vi "QuadRotor_Monitoring_LV1.vi"() -> ()   [LabVIEW 2015]
uses:
  <vilib>/Instr/_visa.llb/VISA Set IO Buffer Mask.ctl
  <vilib>/Instr/_visa.llb/VISA Configure Serial Port (Instr).vi
panel:
  in  "Lontitude_W3":i32=1005738310
  in  "Latitude_W3":i32=139458720
  in  "Lontitude_W2":i32=1005738310
  in  "Latitude_W2":i32=139458720
  in  "Lontitude_W1":i32=1005738310
  in  "Latitude_W1":i32=139458720
  in  "Lon_home":i32=1005748870
  in  "Lat_home":i32=139456050
  out "(GPS_numSat)":u16
  out "return count 2":u32
  out "Roob":i32
  out "Altitude_(Auto)":ext format="%#_3g"
  in  "Set_Altitude_(Auto)":dbl=2.5
  out "string":string
  out "Mode":ext format="%.2f"
  out "Altitude":dbl(slide) scale=0.0..20.0
  out "Altitude":ext format="%.2f"
  out "Yaw":dbl(knob) scale=-180.0..180.0
  out "Pitch":dbl(knob) scale=-90.0..90.0
  out "Roll":dbl(knob) scale=-90.0..90.0
  in  "Write to Quad":bool
  out "Header_58":u8
  out "GPS_Longtitude":ext format="%#.7f"
  out "Pitch":ext format="%.2f"
  out "Yaw":ext format="%.2f"
  out "GPS_Latitude":ext format="%#.7f"
  out "Roll":ext format="%.2f"
  out "return count":u32
  in  "stop":bool
  in  "VISA Serial Data":refnum<visa-resource-name>
  # "Quad Rotor Monitoring and Control with GPS Waypoint"
  # "Data Write to Autonomous Quad Rotor (LAT 9 Point), (LON 10 Point) with Google Map tracking Navigator"
  # "Ex  13.8591411 = 138591411 , 100.5231704 = 1005231704 Using in integer  I32"
  # "9 Point"
  # "10 Point"
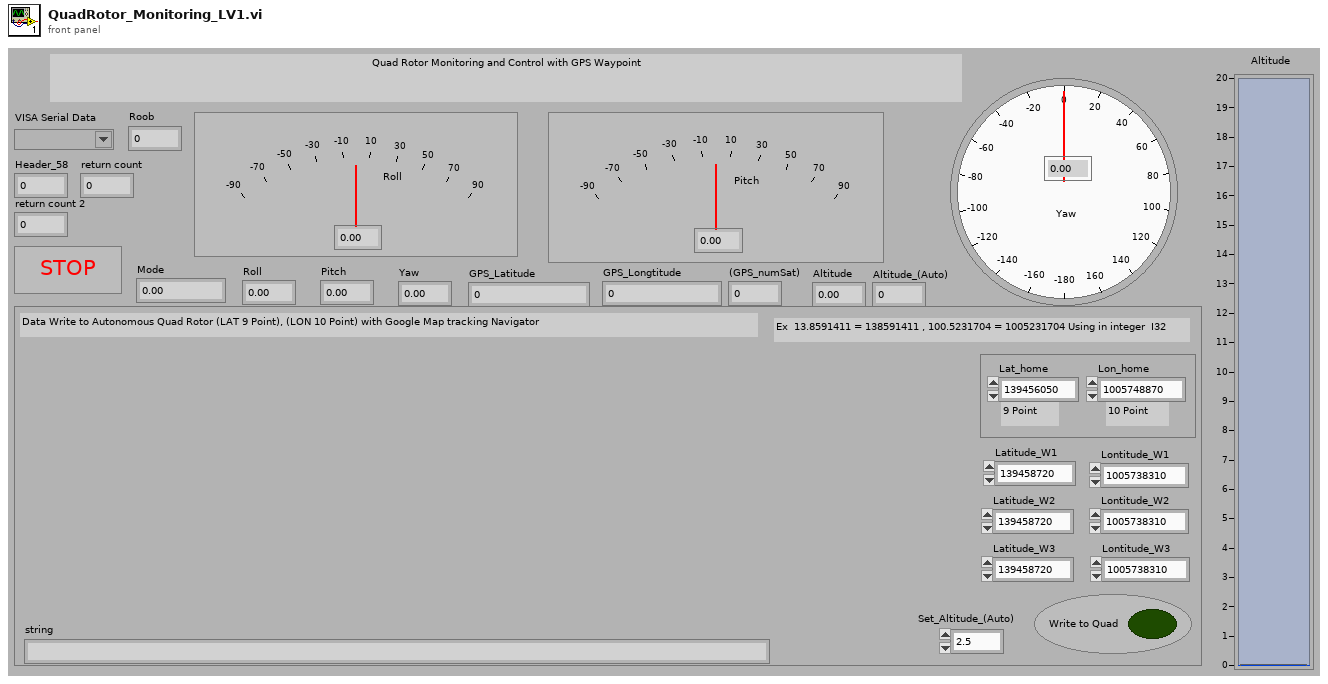
[diagram p1: front panel]
types:
  T1 = typedef "VISA Set IO Buffer Mask.ctl" = u16
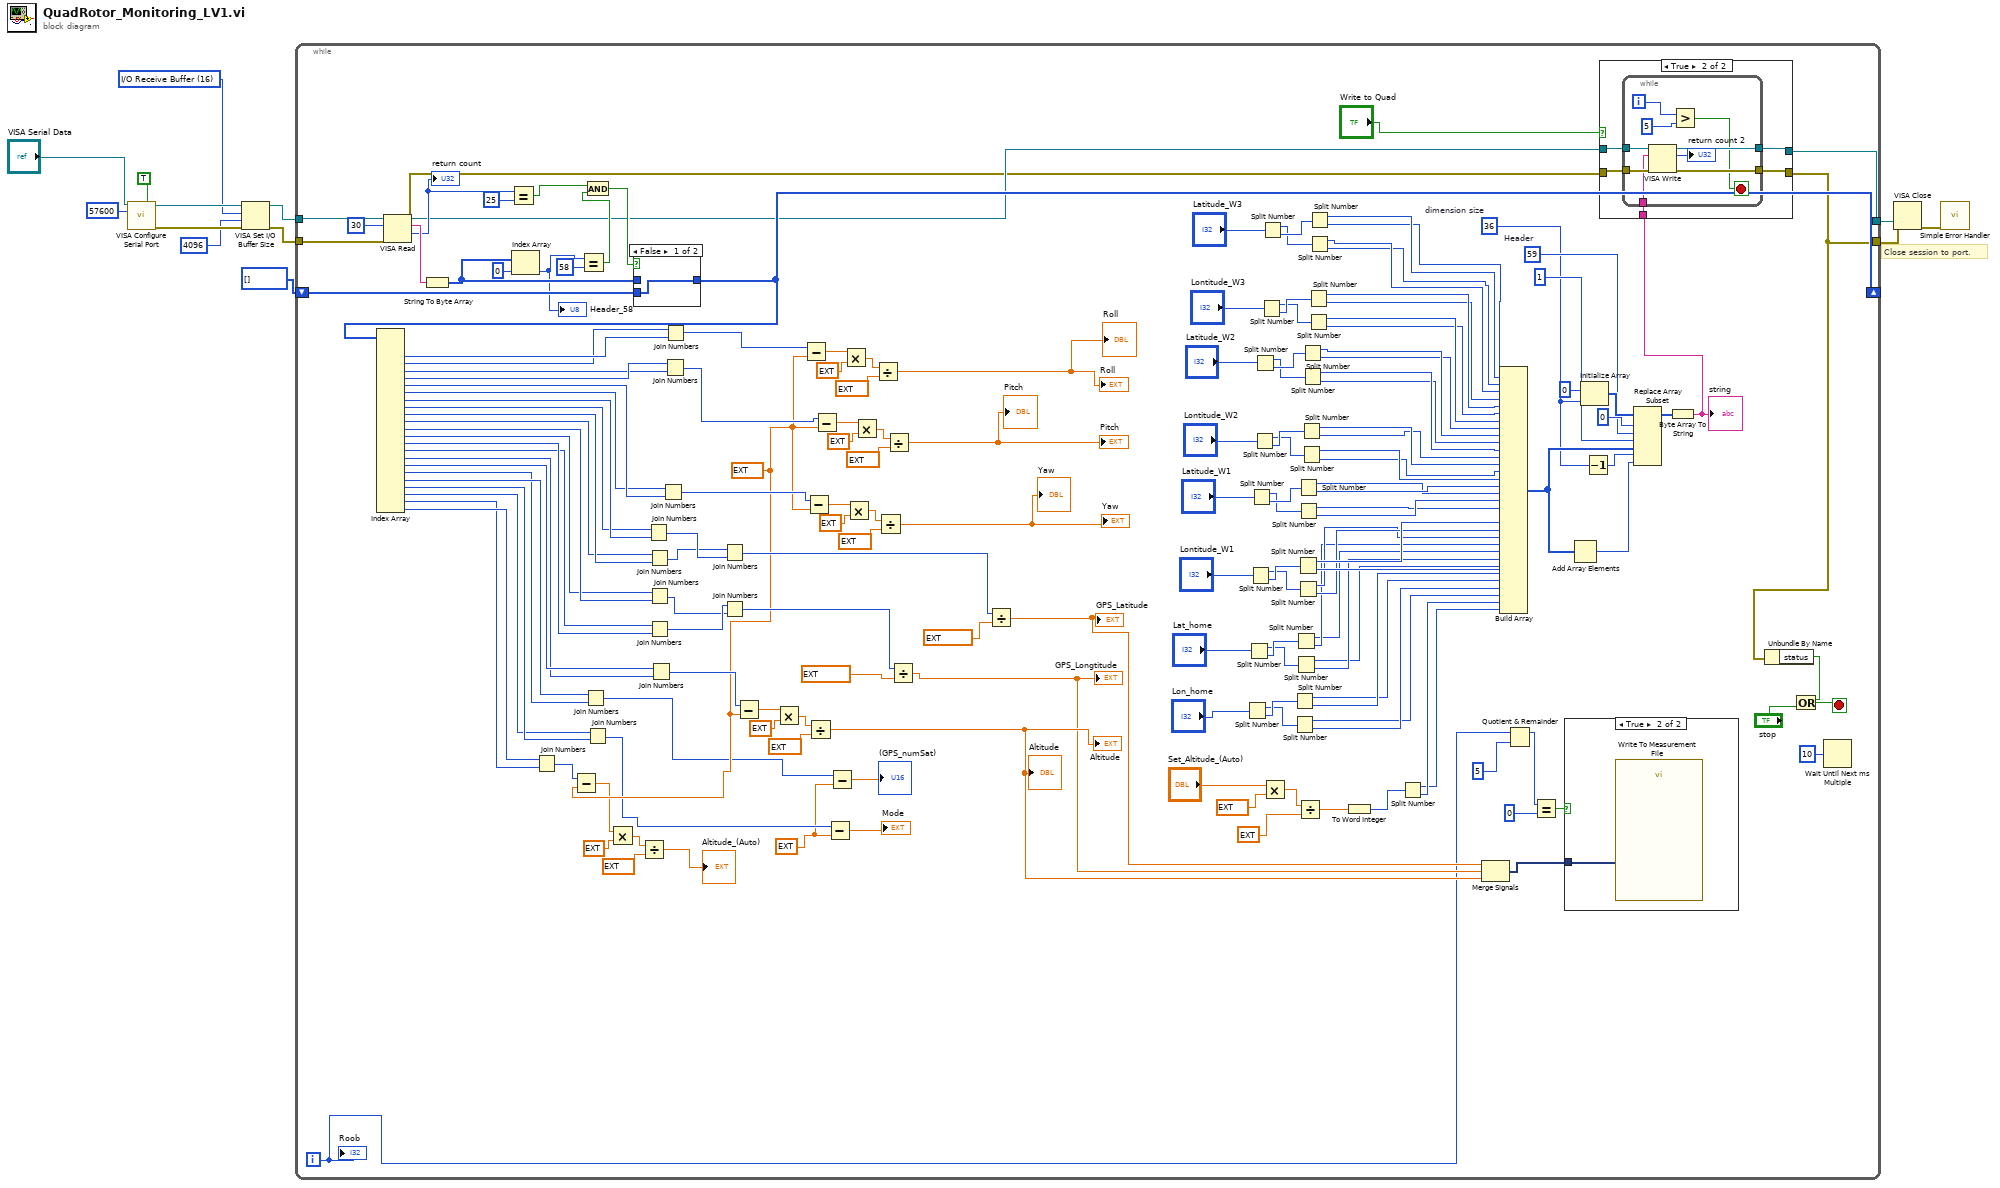
[diagram p0: block diagram]
diagram:
  w10 = T1 16 items=["I/O Receive Buffer"=16, "I/O Transmit Buffer"=32, "I/O Receive and Transmit Buffer"=48] ("Mask")
  # "Close session to port."
  n1 = call-poly "VISA Configure Serial Port"("VISA resource name"="VISA Serial Data", "Enable Termination\nChar (T)"=TRUE ("Enable Termination\nChar (T)"), "baud rate (9600)"=u32 57600) -> ("VISA resource name out"=w12:refnum<visa-resource-name>, "error out"=w11:errorcluster)  [unwired: 7 in, 4 out]
  n2 = VISA Set I/O Buffer Size(VISA resource name=w12, mask (16)=w10, size (4096)=u32 4096, error in (no error)=w11) -> (VISA resource name out=w8:refnum<visa-resource-name>, error out=w6:errorcluster)
  n3 = while {
    tunnel: [w142] -> w7
    tunnel: w8 -> [w183]
    tunnel: [w141] -> w5
    tunnel: w6 -> [w182]
    shift-right: [w152] -> _
    shift-left: u8[] [] ("unsigned byte array") -> [w153]
    i -> [w45]
    stop <- w186 stop-if-true
    w60 = 36  # dimension size
    w109 = u8 59  # Header
    w52 = ext 255.0 ("y")
    w70 = ext 32767.0 ("y")
    n4 = VISA Read(VISA resource name=w183, byte count=u32 30, error in (no error)=w182) -> (VISA resource name out=w144:refnum<visa-resource-name>, read buffer=w156:string, return count=w149:u32, error out=w143:errorcluster)
    "return count" <- w149
    n5 = String To Byte Array(string=w156) -> (unsigned byte array=w154:u8[])
    n6 = Equal?(x=w149, y=u32 25) -> (x = y?=w147:bool)
    n7 = Index Array(array=w154, index=0) -> (element=w146:u8)
    "Header_58" <- w146
    n8 = Equal?(x=w146, y=u8 58) -> (x = y?=w151:bool)
    n9 = And(x=w147, y=w151) -> (x .and. y?=w150:bool)
    n10 = case shown="False" w150 {
      tunnel: w154 -> [_ w205]
      tunnel: [w204 w205] -> w152
      tunnel: w153 -> [w204 _]
      frame False {
      }
      frame True {
      }
    }
    n11 = Index Array(array=w152) -> (element #2=w176:u8, element #3=w175:u8, element #4=w173:u8, element #5=w174:u8, element #6=w180:u8, element #7=w179:u8, element #8=w178:u8, element #9=w177:u8, element #10=w137:u8, element #11=w136:u8, element #12=w133:u8, element #13=w132:u8, element #14=w131:u8, element #15=w130:u8, element #16=w120:u8, element #17=w126:u8, element #18=w118:u8, element #19=w119:u8, element #20=w117:u8, element #21=w116:u8, element #22=w72:u8, element #23=w73:u8)  [unwired: 23 in, 1 out]
    n12 = Join Numbers(hi=w73, lo=w72) -> ((hi.lo)=w71:u16)
    n13 = Subtract(x=w71, y=w70) -> (x-y=w66:ext)
    n14 = Join Numbers(hi=w119, lo=w118) -> ((hi.lo)=w51:u16)
    n15 = Join Numbers(hi=w116, lo=w117) -> ((hi.lo)=w55:u16)
    n16 = Multiply(x=w66, y=ext 100.0) -> (x*y=w68:ext)
    n17 = Divide(x=w68, y=ext 32767.0) -> (x/y=→"Altitude_(Auto)":ext)
    n18 = Join Numbers(hi=w177, lo=w178) -> ((hi.lo)=w135:u16)
    n19 = Join Numbers(hi=w136, lo=w137) -> ((hi.lo)=w134:u16)
    n20 = Join Numbers(hi=w132, lo=w133) -> ((hi.lo)=w114:u16)
    n21 = Join Numbers(hi=w130, lo=w131) -> ((hi.lo)=w115:u16)
    n22 = Join Numbers(hi=w126, lo=w120) -> ((hi.lo)=w121:u16)
    n23 = Join Numbers(hi=w179, lo=w180) -> ((hi.lo)=w162:u16)
    n24 = Join Numbers(hi=w174, lo=w173) -> ((hi.lo)=w157:u16)
    n25 = Join Numbers(hi=w175, lo=w176) -> ((hi.lo)=w171:u16)
    n26 = Join Numbers(hi=w134, lo=w135) -> ((hi.lo)=w139:u32)
    n27 = Join Numbers(hi=w115, lo=w114) -> ((hi.lo)=w129:u32)
    n28 = Subtract(x=w121, y=w70) -> (x-y=w125:ext)
    n29 = Multiply(x=w125, y=ext 100.0) -> (x*y=w123:ext)
    n30 = Subtract(x=w171, y=w70) -> (x-y=w170:ext)
    n31 = Subtract(x=w162, y=w70) -> (x-y=w166:ext)
    n32 = Divide(x=w123, y=ext 32767.0) -> (x/y=w50:ext)
    "Altitude" <- w50
    "Altitude" <- w50
    n33 = Subtract(x=w157, y=w70) -> (x-y=w161:ext)
    n34 = Subtract(x=w55, y=w52) -> (x-y=→"Mode":ext)
    n35 = Subtract(x=w51, y=w52) -> (x-y=→"(GPS_numSat)":ext)
    n36 = Multiply(x=w170, y=ext 180.0) -> (x*y=w168:ext)
    n37 = Multiply(x=w166, y=ext 180.0) -> (x*y=w164:ext)
    n38 = Multiply(x=w161, y=ext 180.0) -> (x*y=w159:ext)
    n39 = Divide(x=w168, y=ext 32767.0) -> (x/y=→"Roll" →"Roll":ext)
    n40 = Divide(x=w164, y=ext 32767.0) -> (x/y=→"Yaw" →"Yaw":ext)
    n41 = Divide(x=w159, y=ext 32767.0) -> (x/y=→"Pitch" →"Pitch":ext)
    n42 = Divide(x=w129, y=ext 10000000.0) -> (x/y=w49:ext)
    "GPS_Longtitude" <- w49
    n43 = Divide(x=w139, y=ext 10000000.0) -> (x/y=w48:ext)
    "GPS_Latitude" <- w48
    n44 = Split Number(x="Lon_home") -> (hi(x)=w102:u16, lo(x)=w103:u16)
    n45 = Split Number(x="Lat_home") -> (hi(x)=w104:u16, lo(x)=w105:u16)
    n46 = Split Number(x="Lontitude_W1") -> (hi(x)=w106:u16, lo(x)=w107:u16)
    n47 = Split Number(x="Latitude_W1") -> (hi(x)=w84:u16, lo(x)=w85:u16)
    n48 = Split Number(x="Lontitude_W2") -> (hi(x)=w40:u16, lo(x)=w41:u16)
    n49 = Split Number(x="Latitude_W2") -> (hi(x)=w38:u16, lo(x)=w39:u16)
    n50 = Split Number(x="Lontitude_W3") -> (hi(x)=w34:u16, lo(x)=w35:u16)
    n51 = Split Number(x="Latitude_W3") -> (hi(x)=w32:u16, lo(x)=w33:u16)
    n52 = Multiply(x="Set_Altitude_(Auto)", y=ext 32767.0) -> (x*y=w76:ext)
    n53 = Split Number(x=w103) -> (hi(x)=w88:u8, lo(x)=w89:u8)
    n54 = Split Number(x=w102) -> (hi(x)=w86:u8, lo(x)=w87:u8)
    n55 = Split Number(x=w105) -> (hi(x)=w92:u8, lo(x)=w93:u8)
    n56 = Split Number(x=w104) -> (hi(x)=w90:u8, lo(x)=w91:u8)
    n57 = Split Number(x=w107) -> (hi(x)=w96:u8, lo(x)=w97:u8)
    n58 = Split Number(x=w106) -> (hi(x)=w94:u8, lo(x)=w95:u8)
    n59 = Split Number(x=w85) -> (hi(x)=w100:u8, lo(x)=w101:u8)
    n60 = Split Number(x=w84) -> (hi(x)=w98:u8, lo(x)=w99:u8)
    n61 = Divide(x=w76, y=ext 100.0) -> (x/y=w74:ext)
    n62 = Split Number(x=w41) -> (hi(x)=w27:u8, lo(x)=w26:u8)
    n63 = Split Number(x=w40) -> (hi(x)=w29:u8, lo(x)=w28:u8)
    n64 = Split Number(x=w39) -> (hi(x)=w23:u8, lo(x)=w22:u8)
    n65 = Split Number(x=w38) -> (hi(x)=w25:u8, lo(x)=w24:u8)
    n66 = Split Number(x=w35) -> (hi(x)=w19:u8, lo(x)=w18:u8)
    n67 = Split Number(x=w34) -> (hi(x)=w21:u8, lo(x)=w20:u8)
    n68 = Split Number(x=w33) -> (hi(x)=w15:u8, lo(x)=w14:u8)
    n69 = Split Number(x=w32) -> (hi(x)=w17:u8, lo(x)=w16:u8)
    n70 = To Word Integer(number=w74) -> (16bit integer=w77:i16)
    n71 = Split Number(x=w77) -> (hi(x)=w78:u8, lo(x)=w79:u8)
    n72 = Merge Signals(w48, w49, w50) -> (w47:dynamicdata)
    n73 = Build Array(w14, w15, w16, w17, w18, w19, w20, w21, w22, w23, w24, w25, w26, w27, w28, w29, w101, w100, w99, w98, w97, w96, w95, w94, w93, w92, w91, w90, w89, w88, w87, w86, w79, w78) -> (w63:u8[])
    n74 = Quotient & Remainder(x=w45, y=u32 5) -> (x-y*floor(x/y)=w42:u32)  [unwired: 1 out]
    n75 = Equal?(x=w42, y=u32 0) -> (x = y?=w44:bool)
    n76 = case shown="True" w44 {
      tunnel: w47 -> [_ w187]
      frame False {
      }
      frame True {
        n77 = call "Write To Measurement File"("Signals"=w187) -> ()  [unwired: 16 in, 3 out]
      }
    }
    n78 = Add Array Elements(numeric array=w63) -> (sum=w62:u8)
    n79 = Initialize Array(u8 0, w60) -> (w113:u8[])
    n80 = Decrement(x=w60) -> (x-1=w61:i32)
    n81 = Replace Array Subset(array=w113, new element #1=w109, index #1=0 ("index"), new element #2=w63, index #2=1 ("index"), new element #3=w62, index #3=w61) -> (w108:u8[])
    n82 = Byte Array To String(unsigned byte array=w108) -> (string=w83:string)
    "string" <- w83
    n83 = case shown="True" "Write to Quad" {
      tunnel: w144 -> [w188 w194]
      tunnel: w143 -> [w189 w191]
      tunnel: [w188 w193] -> w142
      tunnel: [w189 w192] -> w141
      tunnel: w83 -> [_ w190]
      frame False {
      }
      frame True {
        n84 = while {
          tunnel: w194 -> [w203]
          tunnel: [w202] -> w193
          tunnel: [w201] -> w192
          tunnel: w191 -> [w200]
          tunnel: w190 -> [w199]
          i -> [w197]
          stop <- w195 stop-if-true
          n85 = VISA Write(VISA resource name=w203, write buffer=w199, error in (no error)=w200) -> (VISA resource name out=w202:refnum<visa-resource-name>, return count=→"return count 2":u32, error out=w201:errorcluster)
          n86 = Greater?(x=w197, y=5) -> (0:w195:bool)
        }
      }
    }
    n87 = Unbundle By Name(w141) -> ("status"=w184:bool)
    n88 = Or(x=w184, y="stop") -> (x .or. y?=w186:bool)
    n89 = Wait Until Next ms Multiple(millisecond multiple=u32 10) -> ()  [unwired: 1 out]
    "Roob" <- w45
  }
  n90 = VISA Close(VISA resource name=w7, error in (no error)=w5) -> (error out=w9:errorcluster)
  n91 = call <vilib>:"Simple Error Handler.vi"("error in (no error)"=w9) -> ()  [unwired: 1 in, 8 out]
